vi "MDPtrMgr FreeCache.vi"(6 "CacheSize(-1 to Free All caches)":i32=-1, 8 "error in (no error)":errorcluster) -> (0 "error out":errorcluster)   [LabVIEW 2017, in "MDPtr.lvlib"]
uses:
  MDPtr.lvlib
  _MDPtrMgr/MDPtrMgr.lvclass
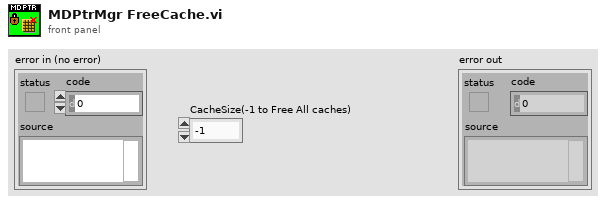
[diagram p1: front panel]
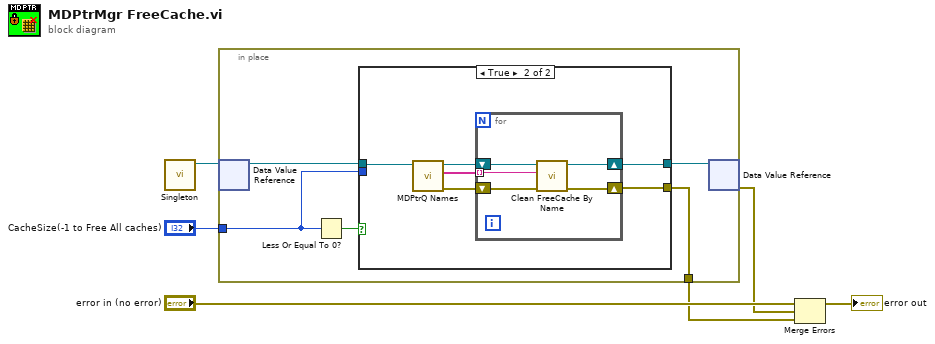
[diagram p0: block diagram]
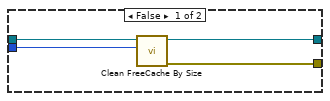
[diagram p2: hidden frame]
diagram:
  n1 = call "Singleton.vi"() -> ("MDPtrMgrDVR"=w4:refnum<data-value>)  [unwired: 9 in, 2 out]
  n2 = in-place {
    in-place-border: "CacheSize(-1 to Free All caches)" -> [w7]
    in-place-border: [w9] -> w1
    n3 = in-place-dvr #1(w4) -> (w11:refnum<class "MDPtrMgr.lvclass">)  [unwired: 1 out]
    n4 = Less Or Equal To 0?(x=w7) -> (x <= 0?=w8:bool)
    n5 = case shown="True" w8 {
      tunnel: w11 -> [w15 w18]
      tunnel: [w14 w17] -> w10
      tunnel: w7 -> [w13 _]
      tunnel: [w12 w16] -> w9
      frame False {
        n6 = call "Clean FreeCache By Size.vi"("CacheSize"=w13, "MDPtrMgr in"=w15) -> ("error out"=w12:errorcluster, "MDPtrMgr out"=w14:refnum<class "MDPtrMgr.lvclass">)  [unwired: 8 in]
      }
      frame True {
        n7 = call "MDPtrQ Names.vi"("MDPtrMgr in"=w18) -> ("error out"=w19:errorcluster, "Queue Names"=w20:string[], "MDPtrMgr out"=w21:refnum<class "MDPtrMgr.lvclass">)  [unwired: 8 in]
        n8 = for {
          tunnel: w20 -> [w22] mode=indexing
          shift-right: [w25] -> w17
          shift-left: w21 -> [w26]
          shift-right: [w23] -> w16
          shift-left: w19 -> [w24]
          n9 = call "Clean FreeCache By Name.vi"("error in (no error)"=w24, "String"=w22, "MDPtrMgr in"=w26) -> ("error out"=w23:errorcluster, "MDPtrMgr out"=w25:refnum<class "MDPtrMgr.lvclass">)  [unwired: 7 in]
        }
      }
    }
    n10 = in-place-dvr #1(w10) -> (w3:errorcluster)  [unwired: 1 out]
  }
  n11 = Merge Errors("error in (no error)", w3, w1) -> (→"error out":errorcluster)
